vi "Log to File.vi"(0 "event data in":T1, 11 "error in":errorcluster) -> (4 "event data out":T1, 15 "error out":errorcluster)   [LabVIEW 2021, in "Event Logger.lvlib"]
uses:
  Event Logger.lvlib
  Converter/Converter Reusables/Converter Reusables.lvlib
  TypeDefs/Event Data Cluster.ctl
  TypeDefs/Event Values.ctl
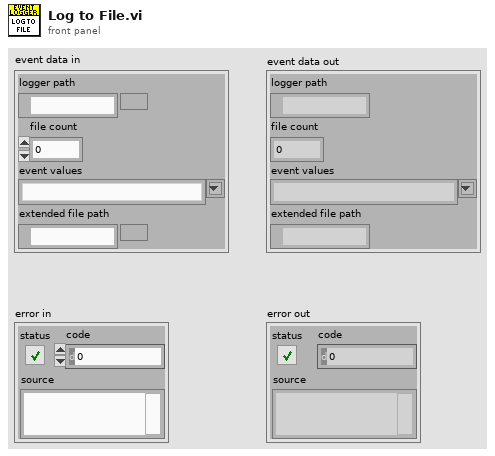
[diagram p1: front panel]
types:
  T1 = typedef "Event Logger.lvlib/Event Data Cluster.ctl" = cluster{"logger path":path, "file count":i32, "event values":T2, "extended file path":path}
  T2 = typedef "Event Logger.lvlib/Event Values.ctl" = string
  T3 = typedef "Converter Reusables.lvlib/Error Information.ctl" = cluster{"subroutine":string, "error data":errorcluster}
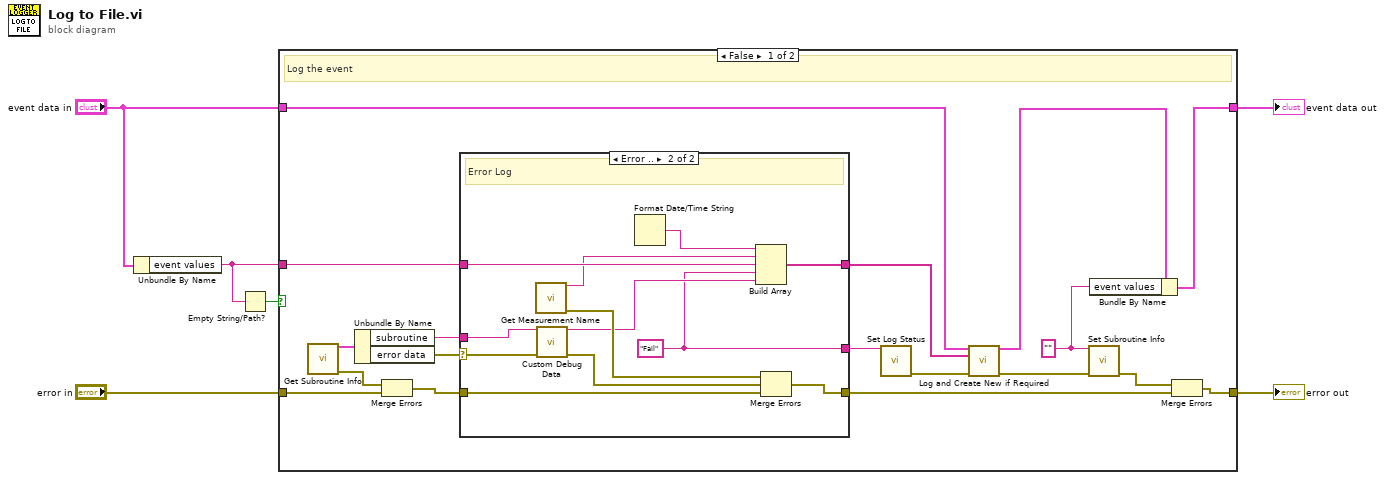
[diagram p0: block diagram]
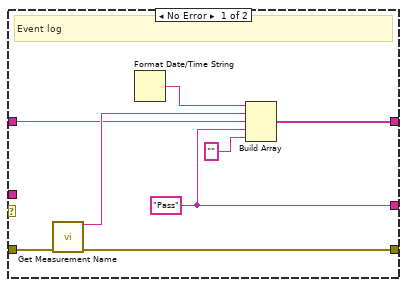
[diagram p2: hidden frame]
diagram:
  n1 = Unbundle By Name("event data in") -> ("event values"=w3:T2)
  n2 = Empty String/Path?(string/path=w3) -> (empty?=w4:bool)
  n3 = case shown="False" w4 {
    tunnel: "error in" -> [w24 w46]
    tunnel: [w11 w46] -> w5
    tunnel: "event data in" -> [w12 w45]
    tunnel: w3 -> [w20 _]
    tunnel: [w7 w45] -> w1
    frame False {
      w8 = "" ("Subroutine In")
      # "Log the event"
      n4 = call "Get Subroutine Info.vi"() -> ("data"=w23:T3, "error out"=w22:errorcluster)  [unwired: 14 in]
      n5 = Unbundle By Name(w23) -> ("subroutine"=w17:string, "error data"=w18:errorcluster)
      n6 = Merge Errors(w22, w24) -> (w21:errorcluster)
      n7 = case shown="Error .." w18 {
        selector: w18 -> [_ w43]
        tunnel: w21 -> [w32 w44]
        tunnel: w20 -> [w29 w40]
        tunnel: [w31 w39] -> w19
        tunnel: [w27 w34] -> w13
        tunnel: w17 -> [_ w42]
        tunnel: [w26 w33] -> w14
        frame No Error {
          w26 = "Pass" ("StatusIn")
          # "Event log"
          n8 = call "Get Measurement Name.vi"("error in"=w32) -> ("name out"=w30:string, "error out"=w31:errorcluster)  [unwired: 13 in]
          n9 = Format Date/Time String() -> (date/time string=w28:string)  [unwired: 3 in]
          n10 = Build Array(w28, w30, w29, w26, "") -> (w27:T2[])
        }
        frame Error {
          w33 = "Fail" ("StatusIn")
          # "Error Log"
          n11 = call "Get Measurement Name.vi"() -> ("name out"=w35:string, "error out"=w37:errorcluster)  [unwired: 14 in]
          n12 = call "Custom Debug Data.vi"("subroutine"=w42, "error in"=w43) -> ("debug info"=w36:string, "error out"=w38:errorcluster)  [unwired: 12 in]
          n13 = Format Date/Time String() -> (date/time string=w41:string)  [unwired: 3 in]
          n14 = Build Array(w41, w35, w40, w33, w36) -> (w34:T2[])
          n15 = Merge Errors(w37, w38, w44) -> (w39:errorcluster)
        }
      }
      n16 = call "Set Log Status.vi"("status in"=w14) -> ("error out"=w16:errorcluster)  [unwired: 14 in]
      n17 = call "Log and Create New if Required.vi"("event data in"=w12, "log data"=w13, "error in"=w16) -> ("event data out"=w9:T1, "error out"=w15:errorcluster)  [unwired: 11 in]
      n18 = call "Set Subroutine Info.vi"("subroutine in"=w8, "error in"=w15) -> ("error out"=w10:errorcluster)  [unwired: 13 in]
      n19 = Bundle By Name(cluster=w9, "event values"=w8) -> (w7:T1)
      n20 = Merge Errors(w10, w19) -> (w11:errorcluster)
    }
    frame True {
      # "Skip logging activity if the event value is empty"
    }
  }
  "error out" <- w5
  "event data out" <- w1
